vi "Power_relay_sw..vi"(8 "error in (no error)":errorcluster {"code" format="%.0x"}, 9 "Power supply setup parameters":T1={"Converter com port"="COM13", "Chroma AC supply GPIB Address"="30", "Conv box used?"=TRUE, "DC Supply GPIB Address"="29"}, 10 "Relay array in":bool[](array[boolean])=[FALSE, FALSE, FALSE, FALSE, FALSE, FALSE, FALSE, FALSE, FALSE, FALSE, FALSE, FALSE, TRUE, FALSE, FALSE], 11 "resource name":refnum<k15>="R_power") -> (0 "error out 2":errorcluster caption="error out" {"code" format="%.0x"})   [LabVIEW 2013]
uses:
  <instrlib>/niSwitch/niSwitch.LLB/niSwitch Topologies.ctl
panel:
  in  "number of relays":i32=13
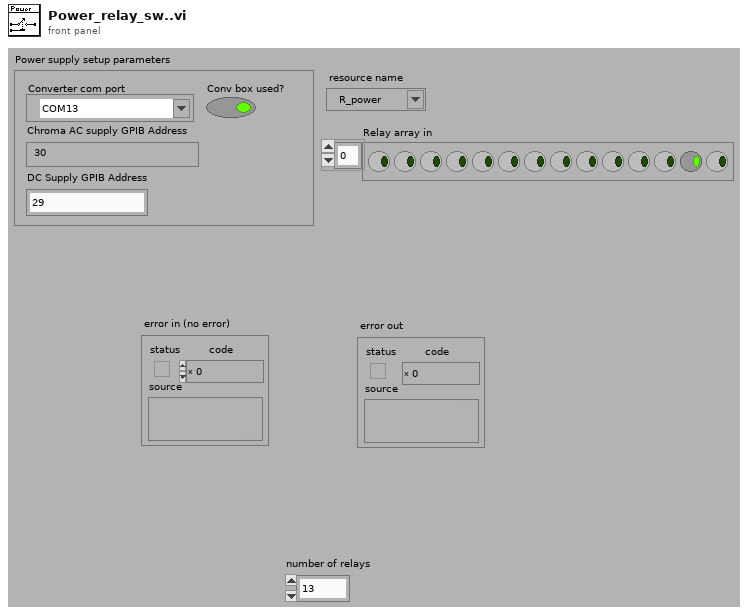
[diagram p1: front panel]
types:
  T1 = cluster{"Converter com port":refnum<visa-resource-name>, "Chroma AC supply GPIB Address":string, "Conv box used?":bool, "DC Supply GPIB Address":string}
  T2 = typedef "niSwitch Topologies.ctl" = string
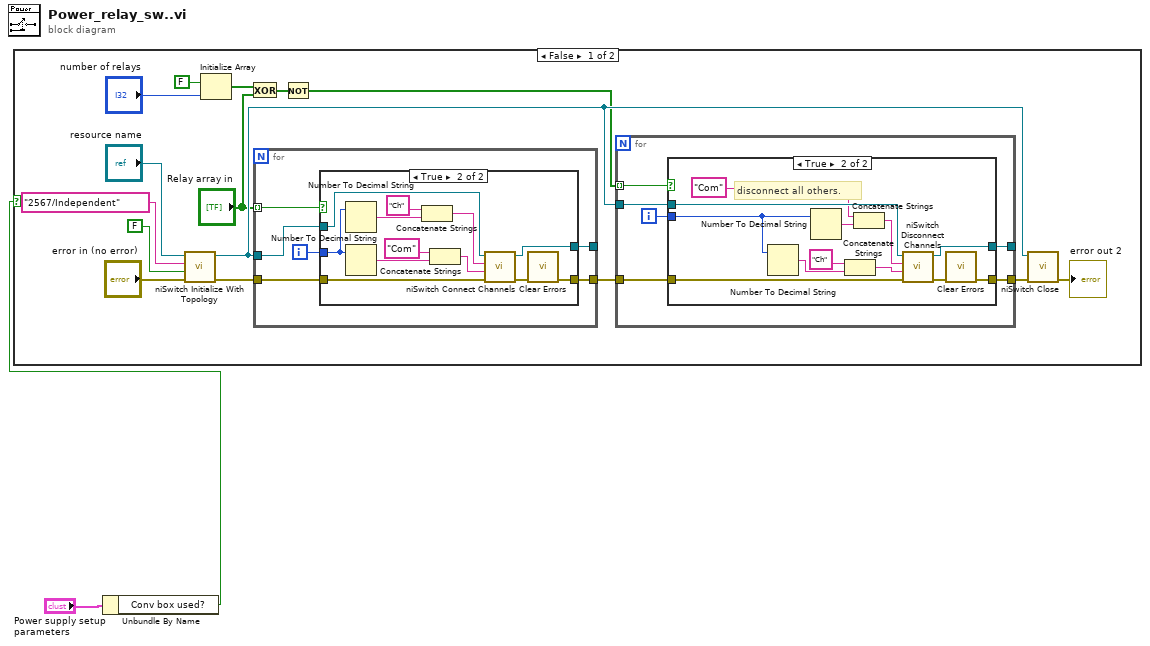
[diagram p0: block diagram]
diagram:
  n1 = Unbundle By Name("Power supply setup parameters") -> ("Conv box used?"=w1:bool)
  n2 = case shown="False" w1 {
    frame False {
      n3 = call <instrlib>:"niSwitch Initialize With Topology.vi"("error in (no error)"="error in (no error)", "reset device (boolean value)"=FALSE, "topology name"=T2 "2567/Independent", "resource name"="resource name") -> ("error out"=w15:errorcluster, "instrument handle out"=w9:refnum<k15>)  [unwired: 6 in]
      n4 = Initialize Array(FALSE ("reset device (boolean value)"), "number of relays") -> (w6:bool[])
      n5 = Exclusive Or(1:"Relay array in", 2:w6) -> (0:w4:bool[])
      n6 = for {
        tunnel: w9 -> [w43]
        tunnel: [w42] -> _
        tunnel: [w41] -> w14
        tunnel: w15 -> [w40]
        tunnel: "Relay array in" -> [w38] mode=indexing
        i -> [w39]
        n7 = case shown="True" w38 {
          tunnel: w43 -> [w45 w57]
          tunnel: [w45 w54] -> w42
          tunnel: [w44 w46] -> w41
          tunnel: w40 -> [w44 w51]
          tunnel: w39 -> [_ w48]
          frame False {
          }
          frame True {
            n8 = Number To Decimal String(number=w48) -> (decimal integer string=w53:string)  [unwired: 1 in]
            n9 = Number To Decimal String(number=w48) -> (decimal integer string=w52:string)  [unwired: 1 in]
            n10 = Concatenate Strings("Ch" ("string"), w53) -> (w56:string)
            n11 = Concatenate Strings("Com" ("string"), w52) -> (w55:string)
            n12 = call <instrlib>:"niSwitch Connect Channels.vi"("error in (no error)"=w51, "channel 2"=w55, "channel 1"=w56, "instrument handle"=w57) -> ("error out"=w47:errorcluster, "instrument handle out"=w54:refnum<k15>)  [unwired: 6 in]
            n13 = call <vilib>:"Clear Errors.vi"("error in (no error)"=w47) -> ("error out"=w46:errorcluster)  [unwired: 6 in]
          }
        }
      }
      n14 = Not(x=w4) -> (.not. x?=w3:bool[])
      n15 = for {
        tunnel: w3 -> [w19] mode=indexing
        tunnel: w9 -> [w23]
        tunnel: [w22] -> _
        tunnel: w14 -> [w21]
        tunnel: [w20] -> w13
        i -> [w18]
        n16 = case shown="True" w19 {
          tunnel: w23 -> [w25 w37]
          tunnel: [w25 w36] -> w22
          tunnel: w21 -> [w24 w35]
          tunnel: [w24 w29] -> w20
          tunnel: w18 -> [_ w26]
          frame False {
          }
          frame True {
            # "disconnect all others."
            n17 = Number To Decimal String(number=w26) -> (decimal integer string=w33:string)  [unwired: 1 in]
            n18 = Number To Decimal String(number=w26) -> (decimal integer string=w32:string)  [unwired: 1 in]
            n19 = Concatenate Strings("Ch" ("string"), w33) -> (w30:string)
            n20 = Concatenate Strings("Com" ("string"), w32) -> (w31:string)
            n21 = call <instrlib>:"niSwitch Disconnect Channels.vi"("error in (no error)"=w35, "channel 2"=w30, "channel 1"=w31, "instrument handle"=w37) -> ("error out"=w34:errorcluster, "instrument handle out"=w36:refnum<k15>)  [unwired: 6 in]
            n22 = call <vilib>:"Clear Errors.vi"("error in (no error)"=w34) -> ("error out"=w29:errorcluster)  [unwired: 6 in]
          }
        }
      }
      n23 = call <instrlib>:"niSwitch Close.vi"("error in (no error)"=w13, "instrument handle"=w9) -> ("error out"=→"error out 2":errorcluster)  [unwired: 9 in]
    }
    frame True {
    }
  }
